vi "Constructor.vi"(8 "error in (no error)":errorcluster, 11 "ChicagoPizzaIngredientFactory in":refnum<class "ChicagoPizzaIngredientFactory.lvclass">) -> (0 "error out":errorcluster, 3 "ChicagoPizzaIngredientFactory out":refnum<class "ChicagoPizzaIngredientFactory.lvclass">)   [LabVIEW 2013, in "ChicagoPizzaIngredientFactory.lvclass"]
uses:
  ChicagoPizzaIngredientFactory.lvclass
  ThickDough.lvclass/ThickDough.lvclass
  PlumTomato.lvclass/PlumTomato.lvclass
  Mozzarella.lvclass/Mozzarella.lvclass
  FrozenClams.lvclass/FrozenClams.lvclass
  ChicagoPizzaIngredientFactory.lvclass/ChicagoPizzaIngredientFactory.ctl
panel:
  # "芝加哥工廠指定芝加哥口味使用的食材"
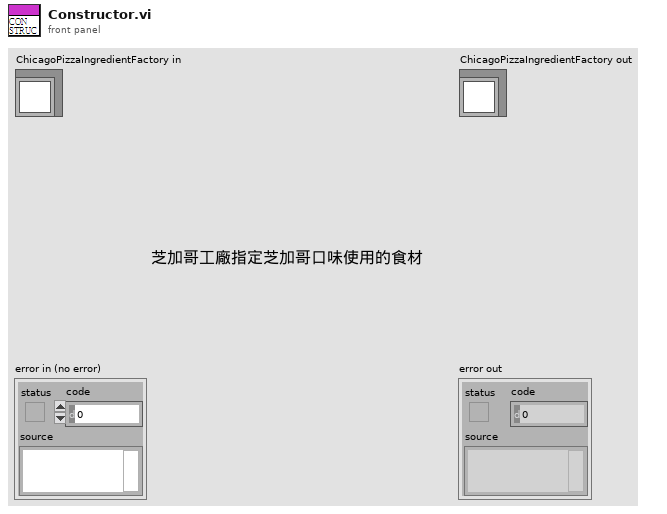
[diagram p1: front panel]
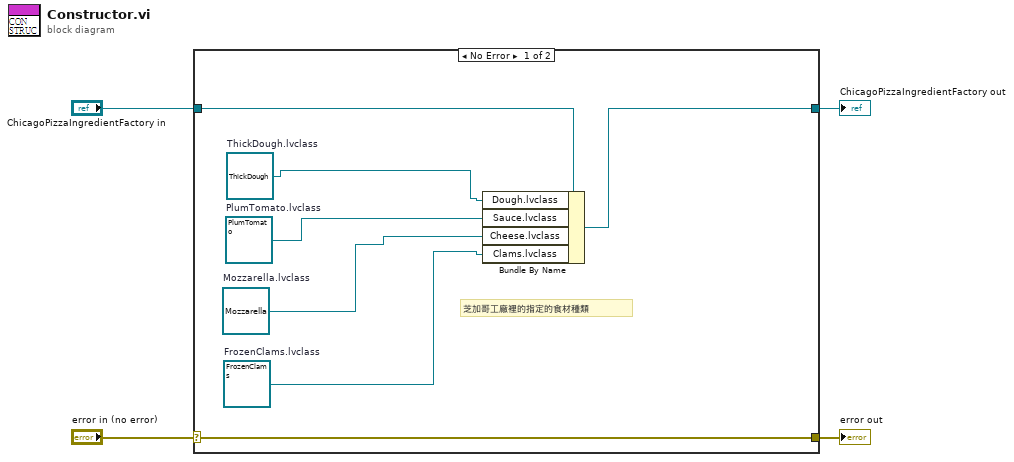
[diagram p0: block diagram]
diagram:
  n1 = case shown="No Error" "error in (no error)" {
    selector: "error in (no error)" -> [w11 w13]
    tunnel: [w11 w13] -> w3
    tunnel: [w9 w12] -> w1
    tunnel: "ChicagoPizzaIngredientFactory in" -> [w10 w12]
    frame No Error {
      w8 = refnum<class "FrozenClams.lvclass"> refnum  # FrozenClams.lvclass
      w7 = refnum<class "Mozzarella.lvclass"> refnum  # Mozzarella.lvclass
      w6 = refnum<class "PlumTomato.lvclass"> refnum  # PlumTomato.lvclass
      w5 = refnum<class "ThickDough.lvclass"> refnum  # ThickDough.lvclass
      # "芝加哥工廠裡的指定的食材種類"
      n2 = Bundle By Name(cluster=w10, "Dough.lvclass"=w5, "Sauce.lvclass"=w6, "Cheese.lvclass"=w7, "Clams.lvclass"=w8) -> (w9:refnum<class "ChicagoPizzaIngredientFactory.lvclass">)
    }
    frame Error {
    }
  }
  "error out" <- w3
  "ChicagoPizzaIngredientFactory out" <- w1
